vi "DAQ_AI_SUM.vi"(5 "error in":errorcluster, 8 "AI Task in":refnum<k21>) -> (0 "error out":errorcluster, 1 "data":dbl format="%0.2f", 3 "AI Task out":refnum<k21>)   [LabVIEW 2025]
uses:
  <vilib>/DAQmx/read.llb/DAQmx Read (Analog 1D DBL 1Chan NSamp).vi
  <vilib>/DAQmx/miscellaneous.llb/DAQmx Fill In Error Info.vi
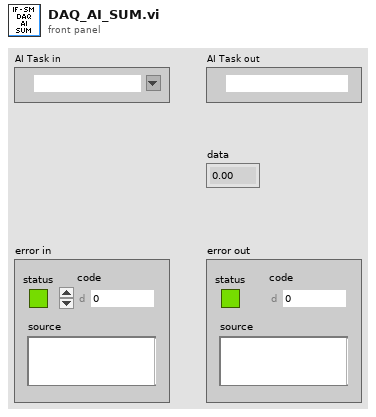
[diagram p1: front panel]
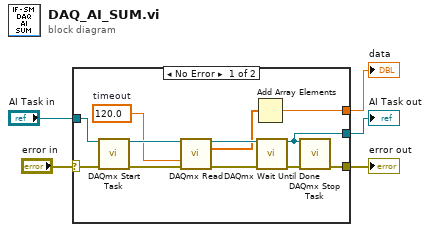
[diagram p0: block diagram]
diagram:
  n1 = case shown="No Error" "error in" {
    selector: "error in" -> [w10 w19]
    tunnel: [w13 w19] -> w5
    tunnel: "AI Task in" -> [w8 w18]
    tunnel: [w9 w18] -> w2
    tunnel: [w6 _] -> w1
    frame No Error {
      w12 = 120.0  # timeout
      n2 = call <vilib>:"DAQmx Start Task.vi"("task/channels in"=w8, "error in"=w10) -> ("task out"=w17:refnum<k21>, "error out"=w15:errorcluster)  [unwired: 12 in]
      n3 = call-poly <vilib>:"DAQmx Read.vi"("task/channels in"=w17, "timeout"=w12, "error in"=w15) -> ("task out"=w16:refnum<k21>, "data"=w7:dbl[], "error out"=w14:errorcluster)  [unwired: 10 in]
      n4 = Add Array Elements(numeric array=w7) -> (sum=w6:dbl)
      n5 = call <vilib>:"DAQmx Wait Until Done.vi"("task/channels in"=w16, "error in"=w14) -> ("task out"=w9:refnum<k21>, "error out"=w11:errorcluster)  [unwired: 12 in]
      n6 = call <vilib>:"DAQmx Stop Task.vi"("task/channels in"=w9, "error in"=w11) -> ("error out"=w13:errorcluster)  [unwired: 12 in, 1 out]
    }
    frame Error {
    }
  }
  "error out" <- w5
  "data" <- w1
  "AI Task out" <- w2
